vi "discrete filter.vi"(9 "R_angvel_raw":sgl, 11 "L_angvel_raw":sgl) -> (0 "R_angvel_filt":sgl, 1 "R_angvel_raw":sgl, 2 "L_angvel_filt":sgl, 3 "L_angvel_raw":sgl)   [LabVIEW 2019]
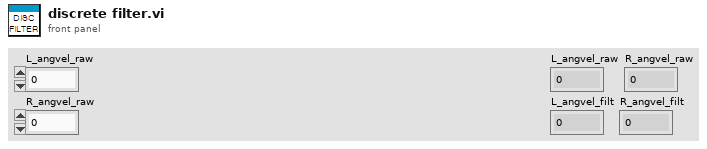
[diagram p1: front panel]
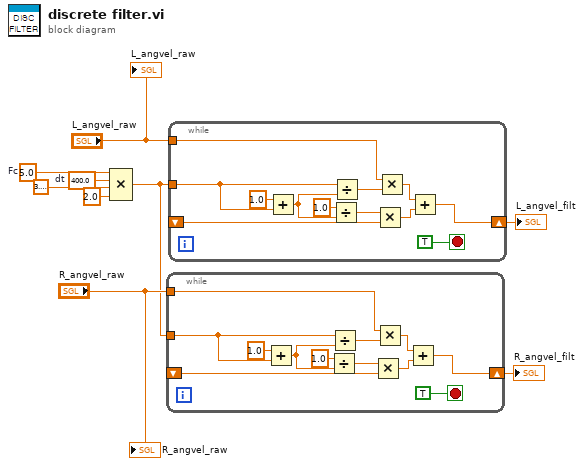
[diagram p0: block diagram]
diagram:
  w7 = sgl 400.0  # dt
  w6 = sgl 5.0  # Fc
  n1 = Compound Arithmetic op=MULTIPLY ("복합 연산")(w6, w7, sgl 3.1415927, sgl 2.0 ("값")) -> (w2:sgl)
  n2 = while {
    tunnel: w2 -> [w10]
    tunnel: "R_angvel_raw" -> [w13]
    shift-right: [w12] -> w1
    shift-left: _ -> [w11]
    stop <- TRUE stop-if-true
    n3 = Add(x=sgl 1.0, y=w10) -> (x+y=w17:sgl)
    n4 = Divide(x=sgl 1.0, y=w17) -> (x/y=w14:sgl)
    n5 = Divide ("나누기")(x=w10, y=w17) -> (x/y=w20:sgl)
    n6 = Multiply(x=w14, y=w11) -> (x*y=w15:sgl)
    n7 = Multiply(x=w13, y=w20) -> (x*y=w16:sgl)
    n8 = Add(x=w16, y=w15) -> (x+y=w12:sgl)
  }
  "R_angvel_filt" <- w1
  n9 = while {
    tunnel: w2 -> [w22]
    tunnel: "L_angvel_raw" -> [w25]
    shift-right: [w24] -> w4
    shift-left: _ -> [w23]
    stop <- TRUE stop-if-true
    n10 = Add(x=sgl 1.0, y=w22) -> (x+y=w29:sgl)
    n11 = Divide(x=sgl 1.0, y=w29) -> (x/y=w26:sgl)
    n12 = Divide ("나누기")(x=w22, y=w29) -> (x/y=w32:sgl)
    n13 = Multiply(x=w26, y=w23) -> (x*y=w27:sgl)
    n14 = Multiply(x=w25, y=w32) -> (x*y=w28:sgl)
    n15 = Add(x=w28, y=w27) -> (x+y=w24:sgl)
  }
  "L_angvel_filt" <- w4
  "L_angvel_raw" <- "L_angvel_raw"
  "R_angvel_raw" <- "R_angvel_raw"
